vi "Read Global Error Manager Spawned flag.vi"(8 "error in (no error)":errorcluster, 11 "Error Manager in":refnum<class "Local Error Manager.lvclass">) -> (0 "error out":errorcluster, 2 "Status":bool, 3 "Error Manager out":refnum<class "Local Error Manager.lvclass">)   [LabVIEW 2020, in "TALOS.lvlib" / "Error Manager.lvlib" / "Local Error Manager.lvclass"]
uses:
  Error Manager.lvclass/Error Manager.ctl
  Local Error Manager/Local Error Manager.lvclass
  Local Error Manager/Local Error Manager.lvclass/Local Error Manager.ctl
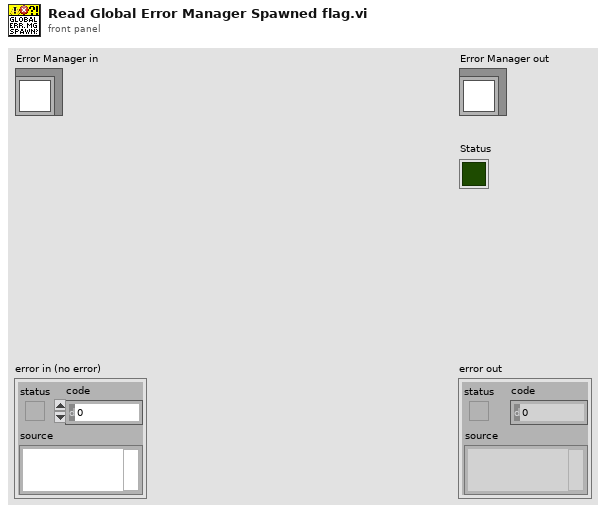
[diagram p1: front panel]
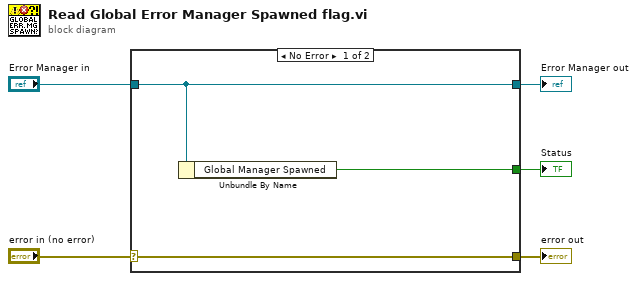
[diagram p0: block diagram]
diagram:
  n1 = case shown="No Error" "error in (no error)" {
    selector: "error in (no error)" -> [w8 w9]
    tunnel: [w8 w9] -> w4
    tunnel: [w7 w10] -> w2
    tunnel: "Error Manager in" -> [w7 w10]
    tunnel: [w6 _] -> w1
    frame No Error {
      n2 = Unbundle By Name(w7) -> ("Global Manager Spawned"=w6:bool)
    }
    frame Error {
    }
  }
  "error out" <- w4
  "Error Manager out" <- w2
  "Status" <- w1
